vi "Match Bots.vi"(8 "Error In":errorcluster, 10 "isRed":bool, 11 "Image Objects":T1) -> (0 "Error Out":errorcluster)   [LabVIEW 2018]
uses:
  Image Object.ctl
  <vilib>/vision/Pattern Matching.llb/IMAQ Curve Parameters.ctl
  Blue Team Data.vi
  Red Team Data.vi
  <vilib>/vision/NI_Vision_Development_Module.lvlib
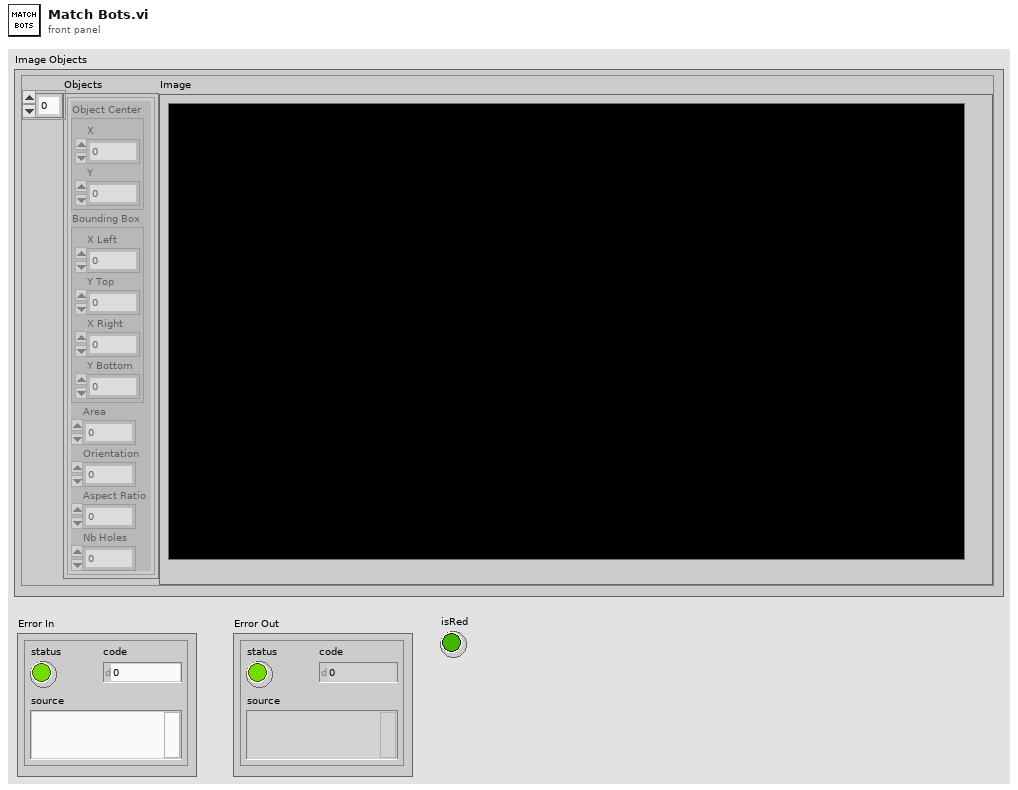
[diagram p1: front panel]
types:
  T1 = typedef "Image Object.ctl" = cluster{"Objects":cluster{"Object Center":cluster{"X":sgl, "Y":sgl}, "Bounding Box":cluster{"X Left":i32, "Y Top":i32, "X Right":i32, "Y Bottom":i32}, "Area":sgl, "Orientation":sgl, "Aspect Ratio":sgl, "Nb Holes":i32}[], "Image":T2}
  T2 = typedef "IMAQ Image.ctl" = refnum<image>
  T3 = cluster{"Object Center":cluster{"X":sgl, "Y":sgl}, "Bounding Box":cluster{"X Left":i32, "Y Top":i32, "X Right":i32, "Y Bottom":i32}, "Area":sgl, "Orientation":sgl, "Aspect Ratio":sgl, "Nb Holes":i32}[]
  T4 = cluster{"Rotation":bool, "Scale":bool, "Occlusion":bool, "Reserved":bool, "Reserved":bool, "Reserved":bool}
  T5 = typedef "IMAQ Curve Parameters.ctl" = cluster{"Extraction Mode":u32, "Edge Threshold":i32, "Edge Filter Size":u32, "Min Length":i32, "Row Search Step Size":i32, "Col Search Step Size":i32, "Max Endpoint Gap":i32, "Closed":bool, "Subpixel":bool}
  T6 = cluster{"X Left":i32, "Y Top":i32, "X Right":i32, "Y Bottom":i32}
  T7 = typedef "IMAQ GM Match Report.ctl" = cluster{"Position":cluster{"x":sgl, "y":sgl}, "Angle":sgl, "Scale":sgl, "Score":sgl, "Bounding Box":cluster{"x":sgl, "y":sgl}[], "Contrast Reversed":bool, "Occlusion %":sgl, "Template Target Curve Score":sgl, "Target Template Curve Score":sgl, "Correlation Score":sgl}
  T8 = cluster{"Object Center":cluster{"X":sgl, "Y":sgl}, "Bounding Box":cluster{"X Left":i32, "Y Top":i32, "X Right":i32, "Y Bottom":i32}, "Area":sgl, "Orientation":sgl, "Aspect Ratio":sgl, "Nb Holes":i32}
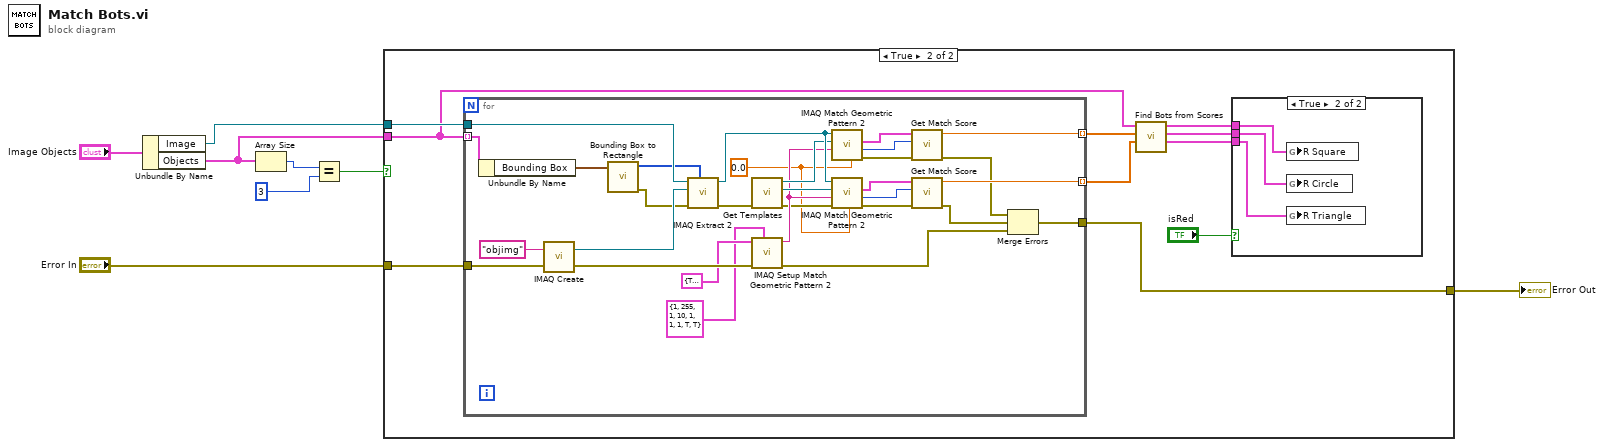
[diagram p0: block diagram]
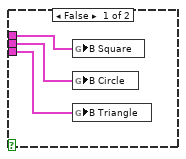
[diagram p3: hidden frame]
diagram:
  n1 = Unbundle By Name("Image Objects") -> ("Image"=w3:T2, "Objects"=w4:T3)
  n2 = Array Size(array=w4) -> (size(s)=w8:i32)
  n3 = Equal?(x=w8, y=3) -> (x = y?=w6:bool)
  n4 = case shown="True" w6 {
    tunnel: w4 -> [_ w15]
    tunnel: w3 -> [_ w19]
    tunnel: "Error In" -> [w9 w18]
    tunnel: [w9 w10] -> w1
    frame False {
    }
    frame True {
      n5 = for {
        tunnel: w15 -> [w51] mode=indexing
        tunnel: w19 -> [w55]
        tunnel: w18 -> [w54]
        tunnel: [w31] -> w17 mode=indexing
        tunnel: [w30] -> w16 mode=indexing
        tunnel: [w26] -> w10
        w38 = sgl 0.0 ("Minimum Match Score")
        n6 = Unbundle By Name(w51) -> ("Bounding Box"=w50:T6)
        n7 = call "IMAQ Create"("Image Name"="objimg", "error in (no error)"=w54) -> ("New Image"=w52:T2, "error out"=w43:errorcluster)  [unwired: 3 in]
        n8 = call "Bounding Box to Rectangle.vi"("Bounding Box"=w50) -> ("Error Out"=w49:errorcluster, "Rectangle"=w48:i32[])  [unwired: 9 in]
        n9 = call "IMAQ Extract 2"("Optional Rectangle"=w48, "error in (no error)"=w49, "Image Dst"=w52, "Image Src"=w55) -> ("error out"=w47:errorcluster, "Image Dst Out"=w46:T2)  [unwired: 6 in]
        n10 = call "Get Templates.vi"("Error In"=w47) -> ("Error Out"=w39:errorcluster, "Circle Template"=w44:T2, "Square Template"=w45:T2)  [unwired: 8 in]
        n11 = call "IMAQ Setup Match Geometric Pattern 2"("Curve Parameters"=T5 {"Extraction Mode"=1, "Edge Threshold"=255, "Edge Filter Size"=1, "Min Length"=10, "Row Search Step Size"=1, "Col Search Step Size"=1, "Max Endpoint Gap"=1, "Closed"=TRUE, "Subpixel"=TRUE}, "error in (no error)"=w43, "Match Mode"=T4 {"Rotation"=TRUE, "Scale"=FALSE, "Occlusion"=FALSE, "Reserved"=TRUE, "Reserved"=FALSE, "Reserved"=FALSE}) -> ("error out"=w27:errorcluster, "Match Geometric Pattern 2 Setup Data"=w40:string)  [unwired: 7 in]
        n12 = call "IMAQ Match Geometric Pattern 2"("Minimum Match Score"=w38, "Match Geometric Pattern 2 Setup Data"=w40, "Template Image"=w45, "Image"=w46) -> ("error out"=w33:errorcluster, "Number of Matches"=w37:i32, "Matches (real-world)"=w36:T7[])  [unwired: 4 in, 1 out]
        n13 = call "IMAQ Match Geometric Pattern 2"("Minimum Match Score"=w38, "error in (no error)"=w39, "Match Geometric Pattern 2 Setup Data"=w40, "Template Image"=w44, "Image"=w46) -> ("error out"=w32:errorcluster, "Number of Matches"=w35:i32, "Matches (real-world)"=w34:T7[])  [unwired: 3 in, 1 out]
        n14 = call "Get Match Score.vi"("Error In"=w33, "Number of Matches"=w37, "Matches (real-world)"=w36) -> ("Error Out"=w29:errorcluster, "Score"=w31:sgl)  [unwired: 6 in, 1 out]
        n15 = call "Get Match Score.vi"("Error In"=w32, "Number of Matches"=w35, "Matches (real-world)"=w34) -> ("Error Out"=w28:errorcluster, "Score"=w30:sgl)  [unwired: 6 in, 1 out]
        n16 = Merge Errors(w29, w28, w27) -> (w26:errorcluster)
      }
      n17 = call "Find Bots from Scores.vi"("Circle Scores"=w16, "Square Scores"=w17, "Bots"=w15) -> ("Triangle"=w11:T8, "Circle"=w12:T8, "Square"=w13:T8)  [unwired: 6 in]
      n18 = case shown="True" "isRed" {
        tunnel: w13 -> [w22 w25]
        tunnel: w12 -> [w21 w24]
        tunnel: w11 -> [w20 w23]
        frame False {
          n19 = global write "Blue Team Data.vi" "B Square"(w22) -> ()
          n20 = global write "Blue Team Data.vi" "B Circle"(w21) -> ()
          n21 = global write "Blue Team Data.vi" "B Triangle"(w20) -> ()
        }
        frame True {
          n22 = global write "Red Team Data.vi" "R Square"(w25) -> ()
          n23 = global write "Red Team Data.vi" "R Circle"(w24) -> ()
          n24 = global write "Red Team Data.vi" "R Triangle"(w23) -> ()
        }
      }
    }
  }
  "Error Out" <- w1
